vi "Poll Control Panel Change.vi"(8 "error in (no error)":errorcluster, 10 "First call?":bool, 11 "Device":refnum<class "Device.lvclass">) -> (0 "error out":errorcluster, 3 "Device out":refnum<class "Device.lvclass">)   [LabVIEW 2015, in "Device.lvclass"]
uses:
  Device.lvclass
  Device.lvclass/Device.ctl
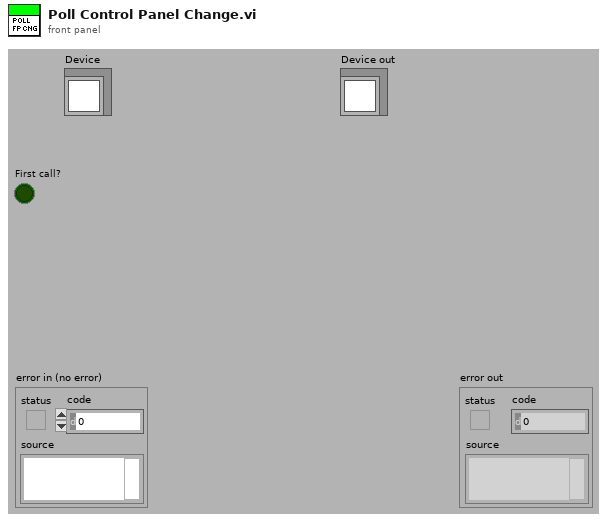
[diagram p1: front panel]
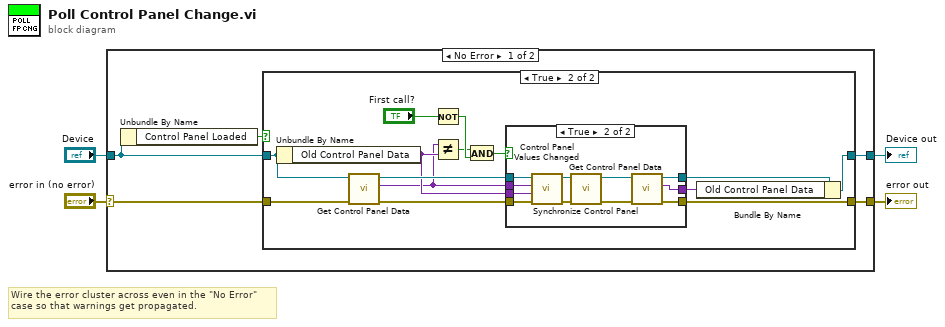
[diagram p0: block diagram]
diagram:
  # "Wire the error cluster across even in the \"No Error\"\ncase so that warnings get propagated."
  n1 = case shown="No Error" "error in (no error)" {
    selector: "error in (no error)" -> [w9 w41]
    tunnel: [w8 w41] -> w2
    tunnel: [w7 w40] -> w3
    tunnel: "Device" -> [w6 w40]
    frame No Error {
      n2 = Unbundle By Name(w6) -> ("Control Panel Loaded"=w5:bool)
      n3 = case shown="True" w5 {
        tunnel: w9 -> [w10 w23]
        tunnel: [w10 w22] -> w8
        tunnel: w6 -> [w11 w17]
        tunnel: [w11 w14] -> w7
        frame False {
        }
        frame True {
          n4 = Unbundle By Name(w17) -> ("Old Control Panel Data"=w15:variant)
          n5 = call-dynamic "Get Control Panel Data.vi"("error in (no error)"=w23, "Device in"=w17) -> ("error out"=w21:errorcluster, "Data"=w13:variant, "Device out"=w20:refnum<class "Device.lvclass">)  [unwired: 7 in]
          n6 = Not(x="First call?") -> (.not. x?=w24:bool)
          n7 = Not Equal?(x=w13, y=w15) -> (x != y?=w19:bool)
          n8 = And(x=w19, y=w24) -> (x .and. y?=w18:bool)
          n9 = case shown="True" w18 {
            tunnel: w21 -> [w28 w39]
            tunnel: w20 -> [w27 w38]
            tunnel: [w28 w31] -> w22
            tunnel: w15 -> [_ w36]
            tunnel: w13 -> [w26 w37]
            tunnel: [w27 w32] -> w16
            tunnel: [w26 w29] -> w12
            frame False {
            }
            frame True {
              n10 = call-dynamic "Control Panel Values Changed.vi"("error in (no error)"=w39, "Old value"=w36, "New value"=w37, "Device in"=w38) -> ("error out"=w34:errorcluster, "Device out"=w35:refnum<class "Device.lvclass">)  [unwired: 6 in]
              n11 = call-dynamic "Synchronize Control Panel.vi"("error in (no error)"=w34, "Device"=w35) -> ("error out"=w30:errorcluster, "Device out"=w33:refnum<class "Device.lvclass">)  [unwired: 8 in]
              n12 = call-dynamic "Get Control Panel Data.vi"("error in (no error)"=w30, "Device in"=w33) -> ("error out"=w31:errorcluster, "Data"=w29:variant, "Device out"=w32:refnum<class "Device.lvclass">)  [unwired: 7 in]
            }
          }
          n13 = Bundle By Name(cluster=w16, "Old Control Panel Data"=w12) -> (w14:refnum<class "Device.lvclass">)
        }
      }
    }
    frame Error {
    }
  }
  "error out" <- w2
  "Device out" <- w3
